vi "read from connection.vi"(8 "error in":errorcluster, 9 "timeout ms (-1)":i32=-1, 11 "connection in":refnum<class "Queue connection.lvclass">) -> (0 "error out":errorcluster, 1 "valid?":bool, 2 "data message":refnum<class "communicator message.lvclass">, 3 "connection out":refnum<class "Queue connection.lvclass">)   [LabVIEW 2015, in "Queue connection.lvclass"]
uses:
  Queue connection.lvclass
  message/communicator message.lvclass
  Queue connection.lvclass/Queue connection.ctl
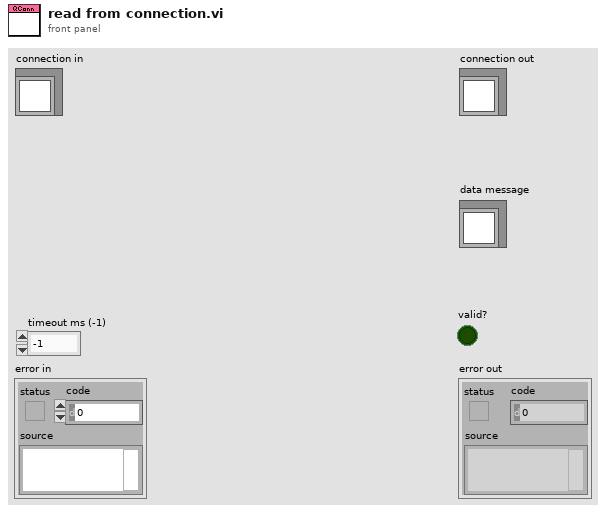
[diagram p1: front panel]
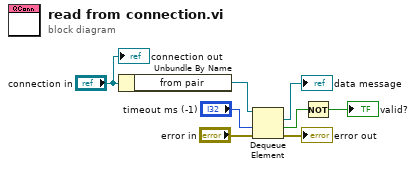
[diagram p0: block diagram]
diagram:
  n1 = Unbundle By Name("connection in") -> ("from pair"=w5:refnum<queue>)
  n2 = Dequeue Element(queue=w5, timeout in ms (-1)="timeout ms (-1)", error in (no error)="error in") -> (element=→"data message":refnum<class "communicator message.lvclass">, timed out?=w2:bool, error out=→"error out":errorcluster)  [unwired: 1 out]
  n3 = Not(x=w2) -> (.not. x?=→"valid?":bool)
  "connection out" <- "connection in"
